vi "Get StringArray.vi"(8 "error in (no error)":errorcluster, 11 "StringArrayMsg in":refnum<class "StringArrayMsg.lvclass">) -> (0 "error out":errorcluster, 2 "Message Data":string[](array[string]), 3 "StringArrayMsg out":refnum<class "StringArrayMsg.lvclass">)   [LabVIEW 2018, in "LapDog.Messaging.v3.NativeArrays.lvlib" / "StringArrayMsg.lvclass"]
doc: "Returns the data contained in the message.\n\nThis method executes regardless of the error in state."
uses:
  StringArrayMsg.lvclass
  StringArrayMsg.lvclass/StringArrayMsg.ctl
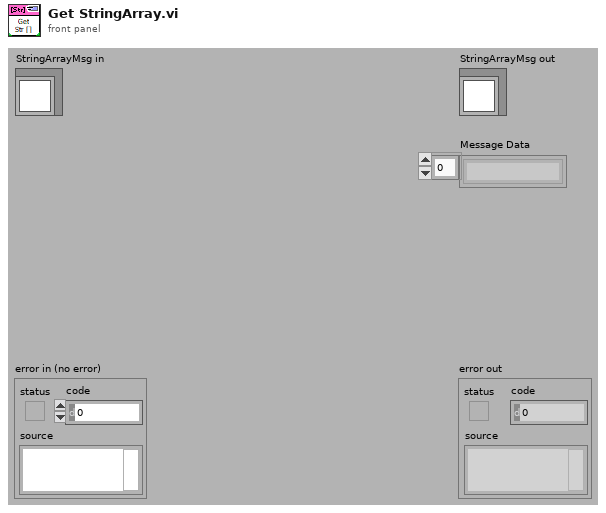
[diagram p1: front panel]
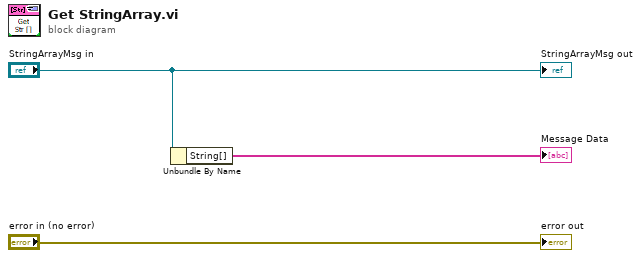
[diagram p0: block diagram]
diagram:
  n1 = Unbundle By Name("StringArrayMsg in") -> ("String[]"=→"Message Data":string[])
  "error out" <- "error in (no error)"
  "StringArrayMsg out" <- "StringArrayMsg in"
